vi "scan2d_prepExperiment.vi"(8 "error in (no error)":errorcluster, 11 "scan_2d in":refnum<class "scan_2d.lvclass">) -> (0 "error out":errorcluster, 3 "scan_2d out":refnum<class "scan_2d.lvclass">)   [LabVIEW 2015, in "scan_2d.lvclass"]
uses:
  scan_2d.lvclass
  scan_2d.lvclass/scan_2d.ctl
  scan_coordinates_tdef.ctl
  <vilib>/Analysis/1siggen.llb/Ramp Pattern by Samples.vi
  <vilib>/Analysis/NI_AALBase.lvlib
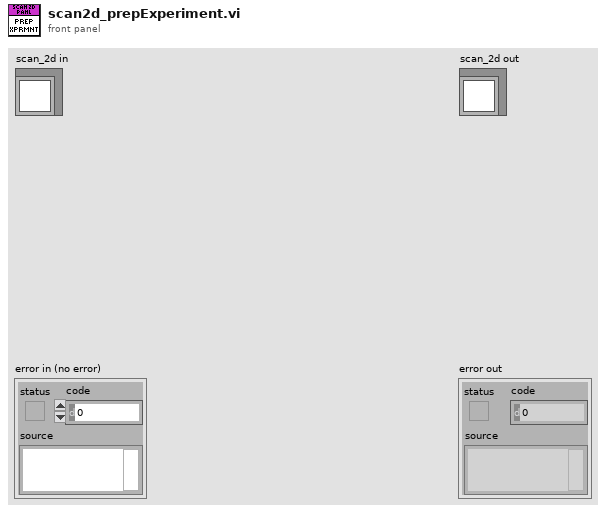
[diagram p1: front panel]
types:
  T1 = typedef "scan_coordinates_tdef.ctl" = cluster{"X":dbl, "Y":dbl, "Retrace?":bool}
  T2 = typedef "scan_2d_stage_settings.ctl" = cluster{"X Start":dbl, "X Stop":dbl, "X Steps":u32, "Y Start":dbl, "Y Stop":dbl, "Y Steps":u32}
  T3 = cluster{"Ramp Pattern":dbl[], "Ramp Pattern":dbl[]}
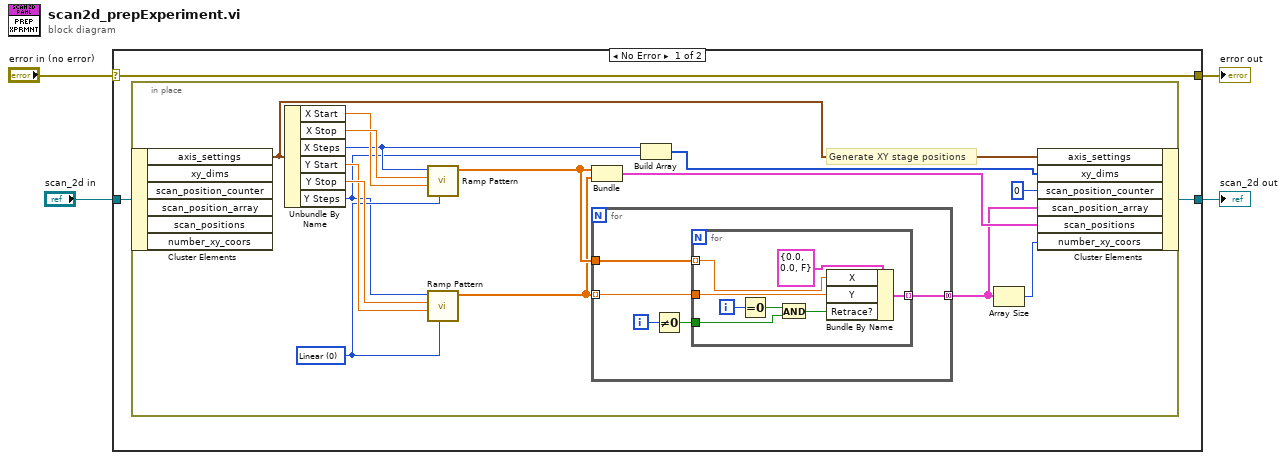
[diagram p0: block diagram]
diagram:
  n1 = case shown="No Error" "error in (no error)" {
    selector: "error in (no error)" -> [w7 w37]
    tunnel: [w7 w37] -> w3
    tunnel: [w5 w36] -> w1
    tunnel: "scan_2d in" -> [w6 w36]
    frame No Error {
      n2 = in-place {
        w18 = u16 0 items=["Linear", "Logarithmic"] ("type")
        # "Generate XY stage positions"
        n3 = in-place-cluster #1(w6) -> ("axis_settings"=w10:T2)  [unwired: 5 out]
        n4 = Unbundle By Name(w10) -> ("X Start"=w21:dbl, "X Stop"=w22:dbl, "X Steps"=w17:u32, "Y Start"=w19:dbl, "Y Stop"=w20:dbl, "Y Steps"=w16:u32)
        n5 = call-poly <vilib>:"Ramp Pattern.vi"("type"=w18, "start"=w21, "end"=w22, "samples"=w17) -> ("Ramp Pattern"=w13:dbl[])  [unwired: 6 in, 1 out]
        n6 = call-poly <vilib>:"Ramp Pattern.vi"("type"=w18, "start"=w19, "end"=w20, "samples"=w16) -> ("Ramp Pattern"=w12:dbl[])  [unwired: 6 in, 1 out]
        n7 = Bundle("Ramp Pattern"=w13, "Ramp Pattern"=w12) -> (w11:T3)  [unwired: 1 in]
        n8 = for {
          tunnel: w12 -> [w26] mode=indexing
          tunnel: w13 -> [w27]
          tunnel: [w25] -> w9 mode=concatenating
          i -> [w24]
          n9 = Not Equal To 0?(x=w24) -> (x != 0?=w23:bool)
          n10 = for {
            tunnel: w27 -> [w35] mode=indexing
            tunnel: w26 -> [w34]
            tunnel: [w33] -> w25 mode=indexing
            tunnel: w23 -> [w29]
            i -> [w31]
            n11 = Equal To 0?(x=w31) -> (x = 0?=w30:bool)
            n12 = And(x=w30, y=w29) -> (x .and. y?=w28:bool)
            n13 = Bundle By Name(cluster=T1 {"X"=0.0, "Y"=0.0, "Retrace?"=FALSE} ("output cluster"), "X"=w35, "Y"=w34, "Retrace?"=w28) -> (w33:T1)
          }
        }
        n14 = Build Array(w17, w16) -> (w15:u32[])
        n15 = Array Size(array=w9) -> (size(s)=w8:i32)
        n16 = in-place-cluster #1("axis_settings"=w10, "xy_dims"=w15, "scan_position_counter"=0, "scan_position_array"=w9, "scan_positions"=w11, "number_xy_coors"=w8) -> (w5:refnum<class "scan_2d.lvclass">)
      }
    }
    frame Error {
    }
  }
  "error out" <- w3
  "scan_2d out" <- w1
